vi "Read subindex.vi"(8 "error in":errorcluster, 11 "EthernetIP Channel in":refnum<class "EthernetIP Channel.lvclass">) -> (0 "error out":errorcluster, 2 "subindex":i32, 3 "EthernetIP Channel out":refnum<class "EthernetIP Channel.lvclass">)   [LabVIEW 2013, in "EthernetIP Channel.lvclass"]
uses:
  EthernetIP Channel.lvclass
  EthernetIP Channel.lvclass/EthernetIP Channel.ctl
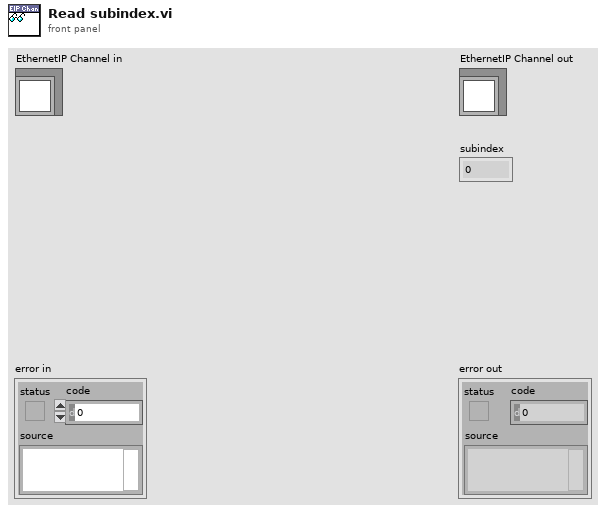
[diagram p1: front panel]
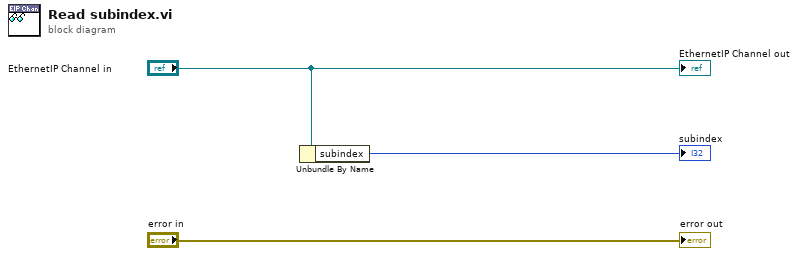
[diagram p0: block diagram]
diagram:
  n1 = Unbundle By Name("EthernetIP Channel in") -> ("subindex"=→"subindex":i32)
  "error out" <- "error in"
  "EthernetIP Channel out" <- "EthernetIP Channel in"
